vi "Configure Gas.vi"(6 "Molbloc Calibration Name (\"\")":string, 7 "Molbloc Calibration Gas (0: Nitrogen)":u16(ring) items=["Nitrogen", "Helium ", "Argon", "Hydrogen", "Oxygen", "Methane", "Ethylene", "Propane", "Ethane", "Butane", "Carbon Monoxide", "Air", "Hexafluoroethane", "Nitrous Oxide", "Carbon Tetrafluoride", "Sulfur Hexafluoride", "Fluoroform", "Carbon Dioxide", "Xenon", "Octofluorocyclobutane"], 8 "error in (no error)":errorcluster, 9 "K Factor (1.0)":dbl=1.0, 10 "Gas Type (0: Nitrogen)":u16(ring) items=["Nitrogen", "Helium", "Argon", "Hydrogen", "Oxygen", "Methane", "Ethylene", "Propane", "Ethane", "Butane", "Carbon Monoxide", "Air", "Hexafluoroethane", "Nitrous Oxide", "Carbon Tetrafluoride", "Sulfur Hexafluoride", "Fluoroform", "Carbon Dioxide", "Xenon", "Octofluorocyclobutane"], 11 "VISA resource name":refnum<visa-resource-name>) -> (0 "error out":errorcluster, 3 "VISA resource name out":refnum<visa-resource-name>)   [LabVIEW 2023, in "Fluke Molbox 1 Plus.lvlib"]
doc: "Sets the gas type that is used for calibration and for flow measurements. This can affect the gas flow coefficient and other measurements."
uses:
  Fluke Molbox 1 Plus.lvlib
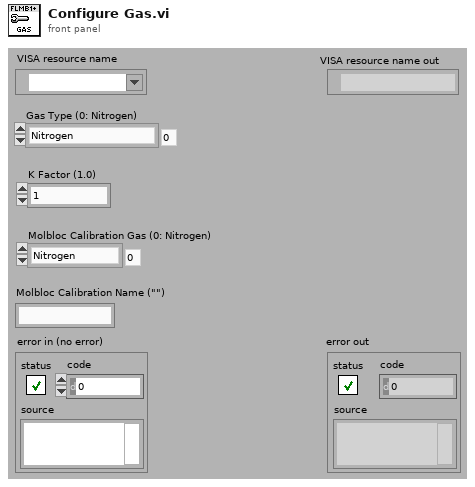
[diagram p1: front panel]
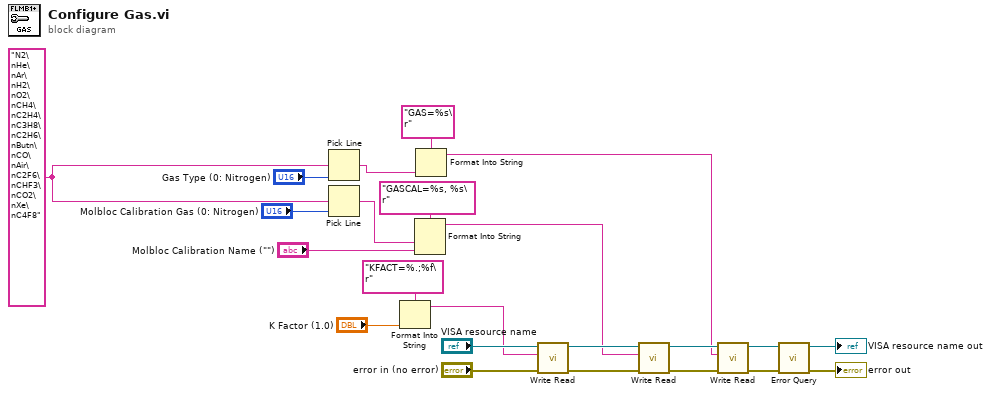
[diagram p0: block diagram]
diagram:
  w19 = "N2\nHe\nAr\nH2\nO2\nCH4\nC2H4\nC3H8\nC2H6\nButn\nCO\nAir\nC2F6\nCHF3\nCO2\nXe\nC4F8" ("multi-line string")
  n1 = Pick Line(multi-line string=w19, line index="Gas Type (0: Nitrogen)") -> (output string=w18:string)  [unwired: 1 in]
  n2 = Pick Line(multi-line string=w19, line index="Molbloc Calibration Gas (0: Nitrogen)") -> (output string=w16:string)  [unwired: 1 in]
  n3 = Format Into String(format string="KFACT=%.;%f\r", "K Factor (1.0)") -> (resulting string=w12:string)  [unwired: 2 in, 1 out]
  n4 = Format Into String(format string="GASCAL=%s, %s\r", w16, "Molbloc Calibration Name (\"\")") -> (resulting string=w9:string)  [unwired: 2 in, 1 out]
  n5 = Format Into String(format string="GAS=%s\r", w18) -> (resulting string=w6:string)  [unwired: 2 in, 1 out]
  n6 = call "Write Read.vi"("error in (no error)"="error in (no error)", "Write String"=w12, "VISA resource name"="VISA resource name") -> ("error out"=w8:errorcluster, "VISA resource name out"=w10:refnum<visa-resource-name>)  [unwired: 6 in, 1 out]
  n7 = call "Write Read.vi"("error in (no error)"=w8, "Write String"=w9, "VISA resource name"=w10) -> ("error out"=w5:errorcluster, "VISA resource name out"=w7:refnum<visa-resource-name>)  [unwired: 6 in, 1 out]
  n8 = call "Write Read.vi"("error in (no error)"=w5, "Write String"=w6, "VISA resource name"=w7) -> ("error out"=w3:errorcluster, "VISA resource name out"=w4:refnum<visa-resource-name>)  [unwired: 6 in, 1 out]
  n9 = call "Error Query.vi"("error in (no error)"=w3, "VISA resource name"=w4) -> ("error out"=→"error out":errorcluster, "VISA resource name out"=→"VISA resource name out":refnum<visa-resource-name>)  [unwired: 6 in, 2 out]
